vi "Read Value.vi"(8 "error in (no error)":errorcluster, 11 "float in":refnum<class "float.lvclass">) -> (0 "error out":errorcluster, 2 "Value":sgl, 3 "float out":refnum<class "float.lvclass">)   [LabVIEW 2020, in "Protobuf RAW.lvlib" / "float.lvclass"]
uses:
  float.lvclass
  float.lvclass/float.ctl
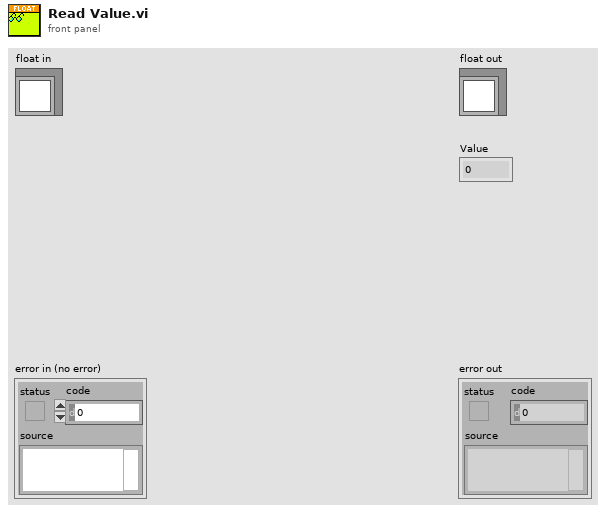
[diagram p1: front panel]
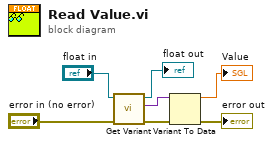
[diagram p0: block diagram]
diagram:
  n1 = call-dynamic "Get Variant.vi"("error in (no error)"="error in (no error)", "Proto Type Common in"="float in") -> ("error out"=w6:errorcluster, "Value"=w2:variant, "Proto Type Common out"=→"float out":refnum<class "float.lvclass">)  [unwired: 7 in]
  n2 = Variant To Data(error in=w6, Variant=w2) -> (data=→"Value":sgl, error out=→"error out":errorcluster)  [unwired: 1 in]
